vi "AutoForwardOrBack.vi"(10 "Case":string, 11 "Drive Speed":dbl) -> ()   [LabVIEW 2016]
uses:
  Robot Global Data.vi
  <vilib>/Rock Robotics/WPI/Utilities/WPI_GetSetVariantRefNum.vi
  <vilib>/Rock Robotics/WPI/RobotDrive/WPI_RobotDriveMecanumDrive_Cartesian.vi
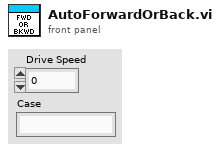
[diagram p1: front panel]
types:
  T1 = typedef "WPI_RobotDriveDevRef.ctl" = cluster{"DevStatus":errorcluster, "Motors[]":T2[], "Square Inputs":bool, "Max Output":dbl}
  T2 = typedef "WPI_MotorControlDeviceRef.ctl" = cluster{"DeviceStatus":errorcluster, "Type":T3, "PWM":cluster{"PWM Channel":T4, "DeadBand":T5}, "CAN":cluster{"Device Number":u8, "SetOutput VI Ref":variant, "GetOutput VI Ref":variant, "Enable VI Ref":variant, "Disable VI Ref":variant, "Data":variant}, "Invert":bool}
  T3 = typedef "WPI_MotorControlType.ctl" = enum16{"PWM", "CAN"}
  T4 = typedef "FPGA_DIOPWMChannel.ctl" = enum8{"PWM 0", "PWM 1", "PWM 2", "PWM 3", "PWM 4", "PWM 5", "PWM 6", "PWM 7", "PWM 8", "PWM 9", "PWM MXP 0", "PWM MXP 1", "PWM MXP 2", "PWM MXP 3", "PWM MXP 4", "PWM MXP 5", "PWM MXP 6", "PWM MXP 7", "PWM MXP 8", "PWM MXP 9", "Invalid"}
  T5 = typedef "WPI_PWMDeadband.ctl" = cluster{"Name":string, "maxPositivePwm":i32, "minPositivePwm":i32, "centerPwm":i32, "maxNegativePwm":i32, "minNegativePwm":i32, "angularRange":u16}
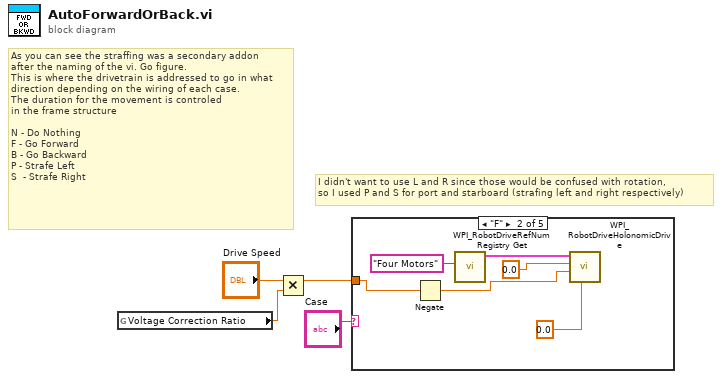
[diagram p0: block diagram]
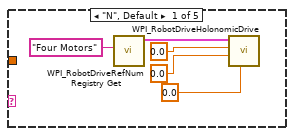
[diagram p2: hidden frame]
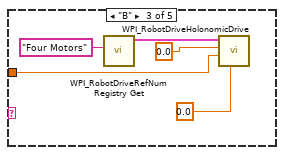
[diagram p3: hidden frame]
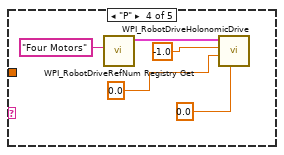
[diagram p4: hidden frame]
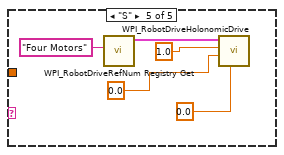
[diagram p5: hidden frame]
diagram:
  # "As you can see the straffing was a secondary addon\nafter the naming of the vi. Go figure.\nThis is where the drivetrain is addressed to go in what\ndirection depending on the wiring of each case.\nThe duration for the movement is controled\nin the frame structure  \n\nN - Do Nothing\nF - Go Forward\nB - Go Backward\nP - Strafe Left\nS  - Strafe Right"
  # "I didn't want to use L and R since those would be confused with rotation,\nso I used P and S for port and starboard (strafing left and right respectively)"
  n1 = global read "Robot Global Data.vi" "Voltage Correction Ratio"() -> (w1:dbl)
  n2 = Multiply(x="Drive Speed", y=w1) -> (x*y=w2:dbl)
  n3 = case shown="\"F\"" "Case" {
    tunnel: w2 -> [_ w11 w18 _ _]
    frame "N", Default {
      n4 = call <vilib>:"WPI_RobotDriveRefNum Registry Get.vi"("refnum name"="Four Motors") -> ("RobotDriveDevRef"=w9:T1)  [unwired: 9 in, 1 out]
      n5 = call-poly <vilib>:"WPI_RobotDriveHolonomicDrive.vi"("Rotation"=0.0, "Y"=0.0, "X"=0.0, "RobotDriveDevRef"=w9) -> ()  [unwired: 5 in, 3 out]
    }
    frame "F" {
      n6 = Negate(x=w11) -> (-x=w10:dbl)
      n7 = call <vilib>:"WPI_RobotDriveRefNum Registry Get.vi"("refnum name"="Four Motors") -> ("RobotDriveDevRef"=w15:T1)  [unwired: 9 in, 1 out]
      n8 = call-poly <vilib>:"WPI_RobotDriveHolonomicDrive.vi"("Rotation"=0.0 ("X"), "Y"=w10, "X"=0.0 ("Y"), "RobotDriveDevRef"=w15) -> ()  [unwired: 5 in, 3 out]
    }
    frame "B" {
      n9 = call <vilib>:"WPI_RobotDriveRefNum Registry Get.vi"("refnum name"="Four Motors") -> ("RobotDriveDevRef"=w20:T1)  [unwired: 9 in, 1 out]
      n10 = call-poly <vilib>:"WPI_RobotDriveHolonomicDrive.vi"("Rotation"=0.0 ("X"), "Y"=w18, "X"=0.0 ("Y"), "RobotDriveDevRef"=w20) -> ()  [unwired: 5 in, 3 out]
    }
    frame "P" {
      n11 = call <vilib>:"WPI_RobotDriveRefNum Registry Get.vi"("refnum name"="Four Motors") -> ("RobotDriveDevRef"=w25:T1)  [unwired: 9 in, 1 out]
      n12 = call-poly <vilib>:"WPI_RobotDriveHolonomicDrive.vi"("Rotation"=0.0 ("X"), "Y"=0.0, "X"=-1.0 ("Y"), "RobotDriveDevRef"=w25) -> ()  [unwired: 5 in, 3 out]
    }
    frame "S" {
      n13 = call <vilib>:"WPI_RobotDriveRefNum Registry Get.vi"("refnum name"="Four Motors") -> ("RobotDriveDevRef"=w30:T1)  [unwired: 9 in, 1 out]
      n14 = call-poly <vilib>:"WPI_RobotDriveHolonomicDrive.vi"("Rotation"=0.0 ("X"), "Y"=0.0, "X"=1.0 ("Y"), "RobotDriveDevRef"=w30) -> ()  [unwired: 5 in, 3 out]
    }
  }
